vi "MHM Set Param.vi"(7 "ulWriteVerify":u32, 8 "error in (no error)":errorcluster, 9 "ulValue":u32, 10 "ulParam":u32, 11 "ulMHMHandle":u32) -> (0 "error out":errorcluster, 3 "function return":u32)   [LabVIEW 2019, in "MHM_1SL_interface.lvlib"]
uses:
  MHM_1SL_interface.lvlib
  lib/MHM_1SL_interface.dll
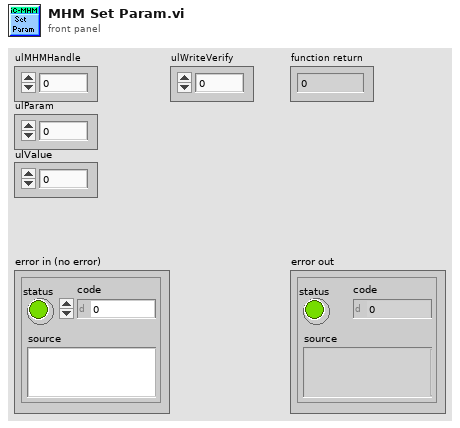
[diagram p1: front panel]
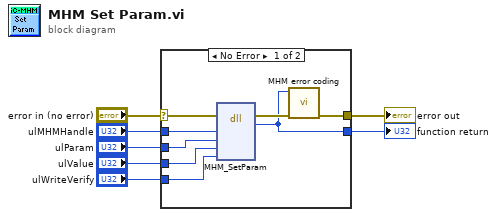
[diagram p0: block diagram]
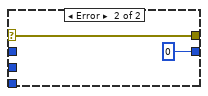
[diagram p2: hidden frame]
diagram:
  n1 = case shown="No Error" "error in (no error)" {
    selector: "error in (no error)" -> [w15 w17]
    tunnel: "ulMHMHandle" -> [w14 _]
    tunnel: "ulParam" -> [w13 _]
    tunnel: "ulValue" -> [w12 _]
    tunnel: "ulWriteVerify" -> [w11 _]
    tunnel: [w9 w17] -> w2
    tunnel: [w8 u32 0] -> w1
    frame No Error {
      n2 = dll-call lib="C:/workspace/project/scancon/MHM_1SL_interface_4.4.0/lv_interface/lib/MHM_1SL_interface.dll" fn="MHM_SetParam"(error in=w15, "ulMHMHandle"=w14, "ulParam"=w13, "ulValue"=w12, "ulWriteVerify"=w11) -> (error out=w10:errorcluster, "return type"=w8:u32)  [unwired: 6 in, 1 out]
      n3 = call "MHM error coding.vi"("error in (no error)"=w10, "function return in"=w8) -> ("error out"=w9:errorcluster)  [unwired: 9 in]
    }
    frame Error {
    }
  }
  "function return" <- w1
  "error out" <- w2
